vi "All_Stages_Aloha.vi"(9 "Aloha":bool, 10 "Stage ID":string) -> (2 "Position Out":dbl[](array[numeric]))   [LabVIEW 2014]
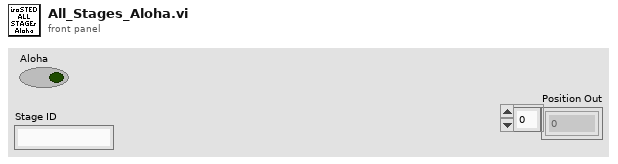
[diagram p1: front panel]
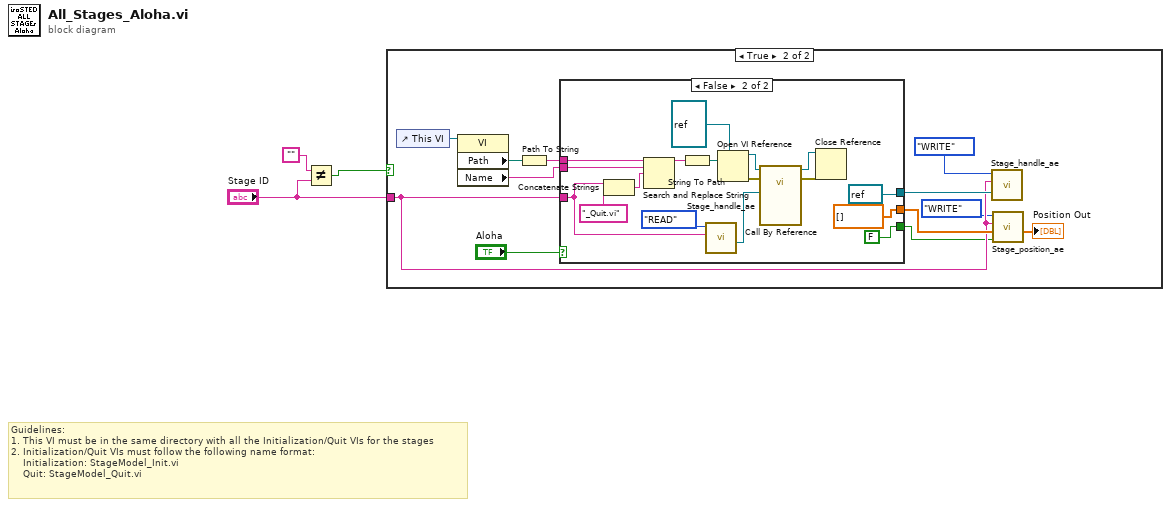
[diagram p0: block diagram]
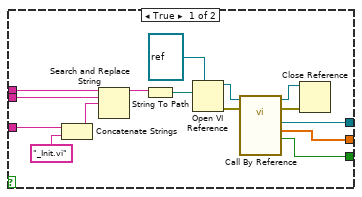
[diagram p3: hidden frame]
diagram:
  # "Guidelines:\n1. This VI must be in the same directory with all the Initialization/Quit VIs for the stages\n2. Initialization/Quit VIs must follow the following name format:\n    Initialization: StageModel_Init.vi\n    Quit: StageModel_Quit.vi"
  n1 = Not Equal?(x="", y="Stage ID") -> (x != y?=w3:bool)
  n2 = case shown="True" w3 {
    tunnel: "Stage ID" -> [_ w7]
    frame False {
    }
    frame True {
      n3 = control-ref of="This VI"() -> (w15:refnum<vi>)
      n4 = property class="VI"(reference=w15) -> ("Path"=w14:path, "Name"=w12:string)  [unwired: 1 in, 2 out]
      n5 = Path To String(path=w14) -> (string=w13:string)
      n6 = case shown="False" "Aloha" {
        tunnel: w13 -> [w30 w47]
        tunnel: w12 -> [w29 w46]
        tunnel: w7 -> [w24 w31]
        tunnel: [w18 refnum<visa-resource-name> refnum ("VISA")] -> w10
        tunnel: [w17 dbl[] [] ("Positions")] -> w9
        tunnel: [w16 FALSE ("Status")] -> w6
        frame True {
          n7 = Concatenate Strings(w24, "_Init.vi" ("string")) -> (w20:string)
          n8 = Search and Replace String(input string=w30, search string=w29, replace string=w20) -> (result string=w28:string)  [unwired: 5 in, 3 out]
          n9 = String To Path(string=w28) -> (path=w27:path)
          n10 = Open VI Reference(type specifier VI Refnum (for type only)=refnum<vi> refnum, vi path=w27) -> (vi reference=w25:refnum<vi>, error out=w22:errorcluster)  [unwired: 4 in]
          n11 = call-by-ref "?"(reference=w25, error in=w22) -> (reference out=w23:refnum<vi>, error out=w21:errorcluster, "Status"=w16:bool, "Position"=w17:dbl[], "VISA Refnum out"=w18:refnum<visa-resource-name>)  [unwired: 9 in]
          n12 = Close Reference(reference=w23, error in (no error)=w21) -> ()  [unwired: 1 out]
        }
        frame False {
          n13 = Concatenate Strings(w31, "_Quit.vi" ("string")) -> (w38:string)
          n14 = Search and Replace String(input string=w47, search string=w46, replace string=w38) -> (result string=w45:string)  [unwired: 5 in, 3 out]
          n15 = String To Path(string=w45) -> (path=w44:path)
          n16 = call "Stage_handle_ae.vi"("StageID"=w31, "Enum"=enum16{"WRITE", "READ"}."READ") -> ("Visa Out"=w32:refnum<visa-resource-name>)  [unwired: 9 in]
          n17 = Open VI Reference(type specifier VI Refnum (for type only)=refnum<vi> refnum, vi path=w44) -> (vi reference=w42:refnum<vi>, error out=w40:errorcluster)  [unwired: 4 in]
          n18 = call-by-ref "?"(reference=w42, error in=w40, "VISA Refnum in"=w32) -> (reference out=w41:refnum<vi>, error out=w39:errorcluster)  [unwired: 11 in]
          n19 = Close Reference(reference=w41, error in (no error)=w39) -> ()  [unwired: 1 out]
        }
      }
      n20 = call "Stage_handle_ae.vi"("VISA In"=w10, "StageID"=w7, "Enum"=enum16{"WRITE", "READ"}."WRITE") -> ()  [unwired: 8 in, 1 out]
      n21 = call "Stage_position_ae.vi"("Status In"=w6, "Position In"=w9, "StageID"=w7, "Enum"=enum16{"WRITE", "READ", "HOME", "SAVE HOME"}."WRITE") -> ("Position Out"=→"Position Out":dbl[])  [unwired: 6 in, 1 out]
    }
  }
